vi "Generate_insert cup locations .vi"(10 "Lifter reading (mm)":dbl, 11 "Select the cup":T1(radio)=enum."Bottom Cup on Beam") -> (1 "Top":dbl, 2 "Middle":dbl, 3 "Bottom":dbl)   [LabVIEW 2019]
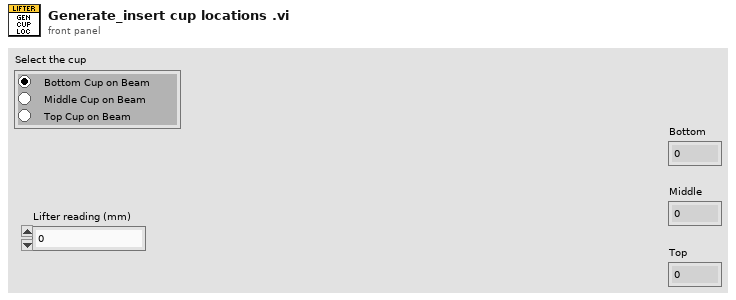
[diagram p1: front panel]
types:
  T1 = enum32{"No Selection", "Bottom Cup on Beam", "Middle Cup on Beam", "Top Cup on Beam"}
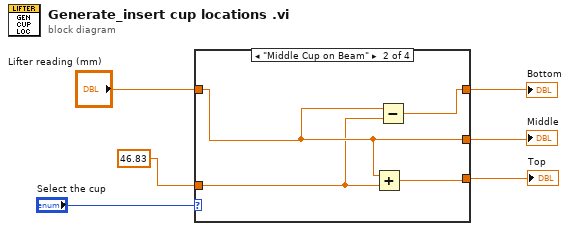
[diagram p0: block diagram]
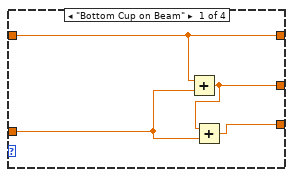
[diagram p2: hidden frame]
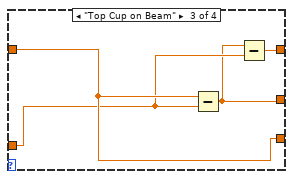
[diagram p3: hidden frame]
diagram:
  n1 = case shown="\"Middle Cup on Beam\"" "Select the cup" {
    tunnel: [w10 w14 w18 _] -> w5
    tunnel: "Lifter reading (mm)" -> [w10 w12 w17 _]
    tunnel: [w9 w12 w15 _] -> w4
    tunnel: [w8 w13 w17 _] -> w3
    tunnel: 46.83 ("y") -> [w7 w11 w16 _]
    frame "Bottom Cup on Beam" {
      n2 = Add(x=w10, y=w7) -> (x+y=w9:dbl)
      n3 = Add(x=w9, y=w7) -> (x+y=w8:dbl)
    }
    frame "Middle Cup on Beam" {
      n4 = Add(x=w12, y=w11) -> (x+y=w13:dbl)
      n5 = Subtract(x=w12, y=w11) -> (x-y=w14:dbl)
    }
    frame "Top Cup on Beam" {
      n6 = Subtract(x=w17, y=w16) -> (x-y=w15:dbl)
      n7 = Subtract(x=w15, y=w16) -> (x-y=w18:dbl)
    }
    frame "No Selection", Default {
    }
  }
  "Bottom" <- w5
  "Middle" <- w4
  "Top" <- w3
